vi "Check Delta Amplitude Extreme bins.vi"(3 "Succ Max Amp":dbl, 4 "Max Difference %":dbl=1.0, 5 "Prev Max Amp":dbl) -> (0 "Check Delta Amp Ok?":bool, 1 "Delta difference %":dbl)   [LabVIEW 2014]
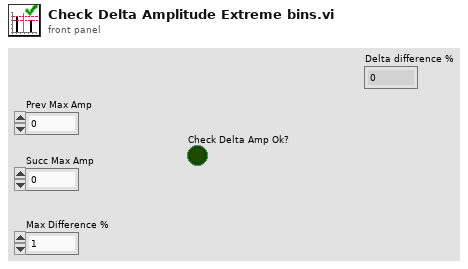
[diagram p1: front panel]
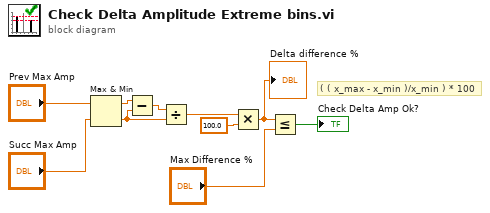
[diagram p0: block diagram]
diagram:
  # "( ( x_max - x_min )/x_min ) * 100"
  n1 = Max & Min(x="Prev Max Amp", y="Succ Max Amp") -> (max(x,y)=w8:dbl, min(x,y)=w6:dbl)
  n2 = Subtract(x=w8, y=w6) -> (x-y=w7:dbl)
  n3 = Divide(x=w7, y=w6) -> (x/y=w5:dbl)
  n4 = Multiply(x=w5, y=100.0) -> (x*y=w3:dbl)
  "Delta difference %" <- w3
  n5 = Less Or Equal?(x=w3, y="Max Difference %") -> (x <= y?=→"Check Delta Amp Ok?":bool)
